vi "getLog.vi"(7 "Offset (0)":i32, 8 "error in (no error)":errorcluster, 9 "Size":i32, 10 "ID in":string, 11 "IDevice in":refnum<class "IDevice.lvclass">) -> (0 "error out":errorcluster, 2 "Log out":string, 3 "IDevice out":refnum<class "IDevice.lvclass">)   [LabVIEW 2022 SP3, in "openDAQ.lvlib" / "IBaseObject.lvlib" / "IPropertyObject.lvlib" / "IComponent.lvlib" / "IFolder.lvlib" / "IDevice.lvlib" / "IDevice.lvclass"]
uses:
  <instrlib>/openDAQ/Public/Classes/IDevice/IDevice.lvclass
  <instrlib>/openDAQ/Public/Classes/IDevice/IDevice.lvclass/IDevice.ctl
  <instrlib>/openDAQ/Public/Classes/daqCoreTypes/IString/IString.lvclass
  <instrlib>/openDAQ/Binaries/Windows/x86/copendaq32.dll
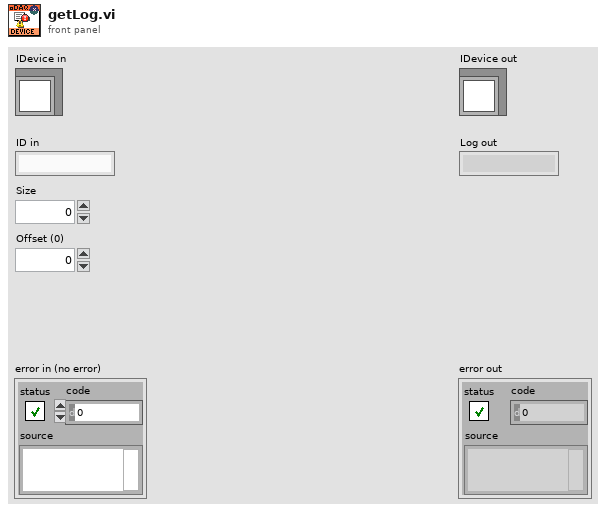
[diagram p1: front panel]
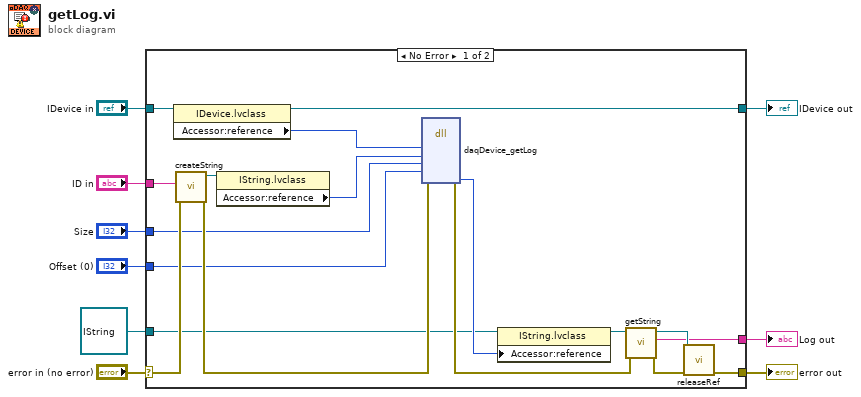
[diagram p0: block diagram]
diagram:
  n1 = case shown="No Error" "error in (no error)" {
    selector: "error in (no error)" -> [w16 w29]
    tunnel: [w20 w29] -> w8
    tunnel: [w25 w28] -> w6
    tunnel: "IDevice in" -> [w27 w28]
    tunnel: refnum<class "IString.lvclass"> refnum ("openDAQ.lvlib:daqCoreTypes.lvlib:IString.lvclass") -> [w14 _]
    tunnel: [w18 _] -> w4
    tunnel: "ID in" -> [w17 _]
    tunnel: "Size" -> [w11 _]
    tunnel: "Offset (0)" -> [w10 _]
    frame No Error {
      n2 = property class="IDevice.lvclass"(reference=w27) -> (reference out=w25:refnum<class "IDevice.lvclass">, "Accessor:reference"=w26:i64)  [unwired: 1 in, 1 out]
      n3 = call <instrlib>:"createString.vi"("error in (no error)"=w16, "String"=w17) -> ("error out"=w15:errorcluster, "IString out"=w13:refnum<class "IString.lvclass">)  [unwired: 8 in]
      n4 = property class="IString.lvclass"(reference=w13) -> ("Accessor:reference"=w12:i64)  [unwired: 1 in, 2 out]
      n5 = dll-call lib="C:/Program Files (x86)/National Instruments/LabVIEW 2022/instr.lib/openDAQ/Binaries/Windows/x86/copendaq*.*" fn="daqDevice_getLog"(error in=w15, "device"=w26, "id"=w12, "size"=w11, "offset"=w10) -> (error out=w22:errorcluster, "log"=w24:i64)  [unwired: 8 in, 1 out]
      n6 = property class="IString.lvclass"(reference=w14, "Accessor:reference"=w24) -> (reference out=w23:refnum<class "IString.lvclass">)  [unwired: 1 in, 1 out]
      n7 = call <instrlib>:"getString.vi"("error in (no error)"=w22, "IString in"=w23) -> ("error out"=w21:errorcluster, "String out"=w18:string, "IString out"=w19:refnum<class "IString.lvclass">)  [unwired: 7 in]
      n8 = call-dynamic "releaseRef.vi"("error in (no error)"=w21, "IBaseObject in"=w19) -> ("error out"=w20:errorcluster)  [unwired: 9 in]
    }
    frame Error {
    }
  }
  "error out" <- w8
  "IDevice out" <- w6
  "Log out" <- w4
